vi "Haversign Function (SubVI).vi"(1 "Set Point Lon (dd)":dbl, 2 "Set Point Lat (dd)":dbl, 3 "Current Lon (dd)":dbl, 4 "Current Lat (dd)":dbl) -> (0 "Separation Distance (m)":dbl)   [LabVIEW 2019]
doc: "Haversign Function - Calculates the distance between two coordinates along a great circle. In this case, earth is idealized as a spheriod with radius of 6372.8 km (based on radius of average circumference). This should be pretty accurate over short distances (such as for a watch circle). \n\nRobert Raye\nNREL 2019"
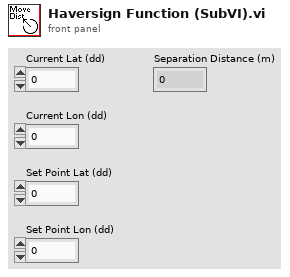
[diagram p1: front panel]
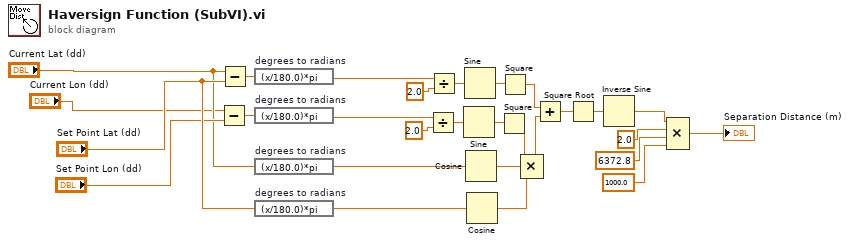
[diagram p0: block diagram]
diagram:
  n1 = Subtract(x="Current Lon (dd)", y="Set Point Lon (dd)") -> (x-y=w2:dbl)
  n2 = Subtract(x="Current Lat (dd)", y="Set Point Lat (dd)") -> (x-y=w1:dbl)
  n3 = expression code="(x/180.0)*pi" "degrees to radians"(w1) -> (w16:dbl)
  n4 = expression code="(x/180.0)*pi" "degrees to radians"(w2) -> (w17:dbl)
  n5 = expression code="(x/180.0)*pi" "degrees to radians"("Current Lat (dd)") -> (w18:dbl)
  n6 = expression code="(x/180.0)*pi" "degrees to radians"("Set Point Lat (dd)") -> (w19:dbl)
  n7 = Divide(x=w17, y=2.0) -> (x/y=w7:dbl)
  n8 = Divide(x=w16, y=2.0) -> (x/y=w4:dbl)
  n9 = Sine(x=w7) -> (sin(x)=w8:dbl)
  n10 = Sine(x=w4) -> (sin(x)=w5:dbl)
  n11 = Cosine(x=w18) -> (cos(x)=w21:dbl)
  n12 = Cosine(x=w19) -> (cos(x)=w20:dbl)
  n13 = Square(x=w8) -> (x^2=w22:dbl)
  n14 = Square(x=w5) -> (x^2=w11:dbl)
  n15 = Compound Arithmetic op=MULTIPLY(w22, w21, w20) -> (w10:dbl)
  n16 = Add(x=w11, y=w10) -> (x+y=w12:dbl)
  n17 = Square Root(x=w12) -> (sqrt(x)=w9:dbl)
  n18 = Inverse Sine(1:w9) -> (0:w23:dbl)
  n19 = Compound Arithmetic op=MULTIPLY(w23, 2.0 ("y"), 6372.8 ("y"), 1000.0 ("value")) -> (→"Separation Distance (m)":dbl)
